vi "level.vi"() -> ()   [LabVIEW 2015]
panel:
  in  "Level":i32
  out "Waveform Graph":dbl[](graph)
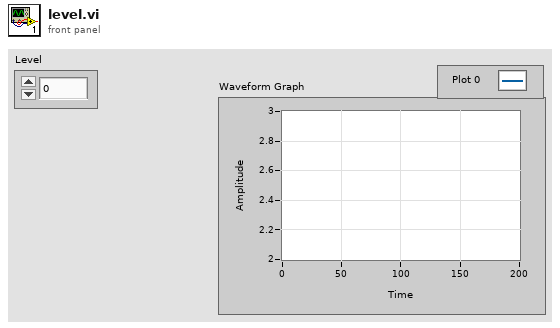
[diagram p1: front panel]
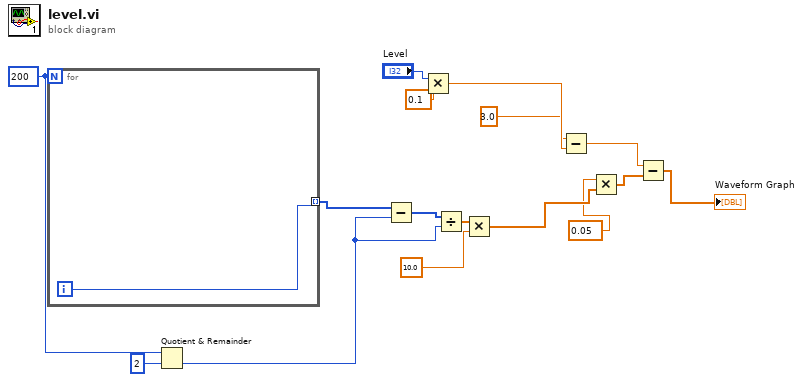
[diagram p0: block diagram]
diagram:
  w15 = 200
  n1 = for {
    N: w15 -> [_]
    tunnel: [w17] -> w16 mode=indexing
    i -> [w17]
  }
  n2 = Quotient & Remainder(x=w15, y=2) -> (floor(x/y)=w12:i32)  [unwired: 1 out]
  n3 = Subtract(x=w16, y=w12) -> (x-y=w13:i32[])
  n4 = Multiply(x="Level", y=0.1) -> (x*y=w7:dbl)
  n5 = Divide(x=w13, y=w12) -> (x/y=w11:dbl[])
  n6 = Multiply(x=w11, y=10.0) -> (x*y=w6:dbl[])
  n7 = Subtract(x=3.0, y=w7) -> (x-y=w3:dbl)
  n8 = Multiply(x=0.05, y=w6) -> (x*y=w4:dbl[])
  n9 = Subtract(x=w3, y=w4) -> (x-y=→"Waveform Graph":dbl[])
